vi "provide_OME_data.vi"(8 "error in (no error)":errorcluster, 9 "image ID":string, 10 "OME element in":refnum<class "XMLElement.lvclass">, 11 "ScanModeTS090821Circular2D in":refnum<class "ImagingModeTS090821Circular2D.lvclass">) -> (0 "error out":errorcluster, 2 "OME element out":refnum<class "XMLElement.lvclass">, 3 "ScanModeTS090821Circular2D out":refnum<class "ImagingModeTS090821Circular2D.lvclass">)   [LabVIEW 2010]
uses:
  common/classes/XMLElement/XMLElement/XMLElement.lvclass
  common/classes/SoftwareParameter/SoftwareParameter/SoftwareParameter.lvclass
  ImagingModeTS090821Circular2D.lvclass
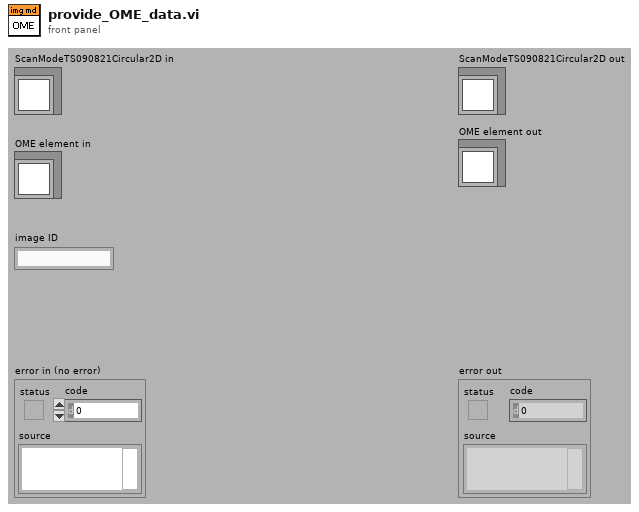
[diagram p1: front panel]
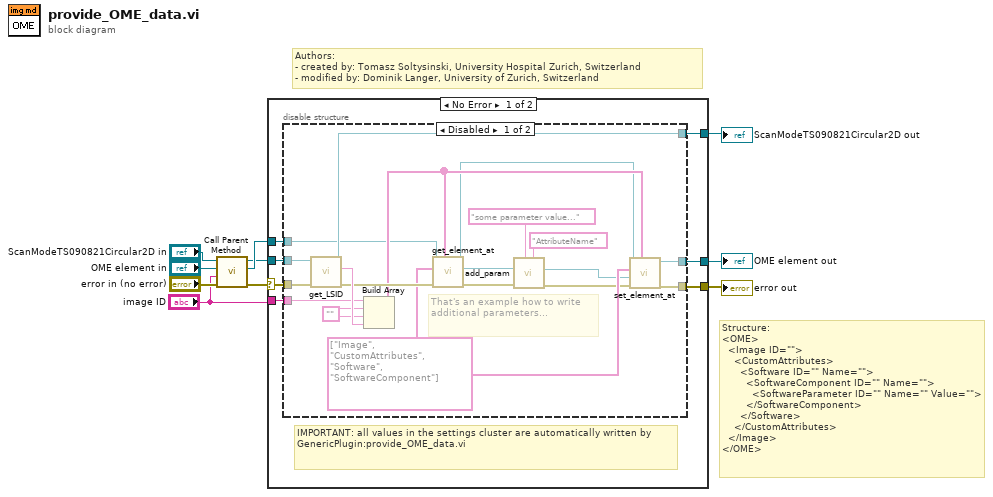
[diagram p0: block diagram]
diagram:
  # "Structure:\n<OME>\n  <Image ID=\"\">\n    <CustomAttributes>\n      <Software ID=\"\" Name=\"\">\n        <SoftwareComponent ID=\"\" Name=\"\">\n          <SoftwareParameter ID=\"\" Name=\"\" Value=\"\">\n        </SoftwareComponent>\n      </Software>\n    </CustomAttributes>\n  </Image>\n</OME>"
  # "Authors: \n- created by: Tomasz Soltysinski, University Hospital Zurich, Switzerland\n- modified by: Dominik Langer, University of Zurich, Switzerland"
  n1 = call-parent "Call Parent Method"("error in (no error)"="error in (no error)", "image ID"="image ID", "OME element in"="OME element in", "ScanModeDL090923Scaffold in"="ScanModeTS090821Circular2D in") -> ("error out"=w7:errorcluster, "OME element out"=w4:refnum<class "XMLElement.lvclass">, "ScanModeDL090923Scaffold out"=w3:refnum<class "ImagingModeTS090821Circular2D.lvclass">)  [unwired: 5 in]
  n2 = case shown="No Error" w7 {
    selector: w7 -> [w16 w40]
    tunnel: w3 -> [w17 w42]
    tunnel: [w12 w41] -> w5
    tunnel: w4 -> [w13 w41]
    tunnel: [w11 w40] -> w1
    tunnel: [w14 w42] -> w2
    tunnel: "image ID" -> [w15 _]
    frame No Error {
      # "IMPORTANT: all values in the settings cluster are automatically written by GenericPlugin:provide_OME_data.vi"
      n3 = disable-structure shown="Disabled" {
        disable-tunnel: w17 -> [w34 w39]
        disable-tunnel: w16 -> [w33 w37]
        disable-tunnel: w15 -> [w32 _]
        disable-tunnel: [w27 w39] -> w14
        disable-tunnel: w13 -> [w26 w38]
        disable-tunnel: [w25 w38] -> w12
        disable-tunnel: [w24 w37] -> w11
        frame Disabled {
          w35 = ""
          w30 = string[] ["Image", "CustomAttributes", "Software", "SoftwareComponent"]
          # "That's an example how to write additional parameters..."
          n4 = call-dynamic "get_LSID.vi"("error in (no error)"=w33, "GenericPlugin in"=w34) -> ("error out"=w31:errorcluster, "LSID (string)"=w36:string, "GenericPlugin out"=w27:refnum<class "ImagingModeTS090821Circular2D.lvclass">)  [unwired: 6 in, 1 out]
          n5 = Build Array(w32, w35, w35, w36) -> (w29:string[])
          n6 = call "get_element_at.vi"("ignore IDs"=w29, "error in (no error)"=w31, "key chain"=w30, "Element in"=w26) -> ("error out"=w21:errorcluster, "element"=w20:refnum<class "XMLElement.lvclass">, "Element out"=w28:refnum<class "XMLElement.lvclass">)  [unwired: 4 in, 1 out]
          n7 = call "add_param.vi"("name"="AttributeName" ("String"), "value"="some parameter value...", "error in (no error)"=w21, "parent element in"=w20) -> ("error out"=w23:errorcluster, "parent element out"=w22:refnum<class "XMLElement.lvclass">)  [unwired: 5 in, 1 out]
          n8 = call "set_element_at.vi"(7:w29, "error in (no error)"=w23, "element"=w22, "key chain"=w30, "Element in"=w28) -> ("error out"=w24:errorcluster, "Element out"=w25:refnum<class "XMLElement.lvclass">)  [unwired: 5 in]
        }
        frame Enabled {
        }
      }
    }
    frame Error {
    }
  }
  "error out" <- w1
  "ScanModeTS090821Circular2D out" <- w2
  "OME element out" <- w5
